vi "Get Test Library Path.vi"(11 "LUnit Test Suite Tests in":refnum<class "LUnit Test Suite Tests.lvclass">) -> (2 "project containing lvlib path":path, 3 "lvlib path":path)   [LabVIEW 2020, in "LUnit Test Suite Tests.lvclass"]
uses:
  LUnit Test Suite Tests.lvclass
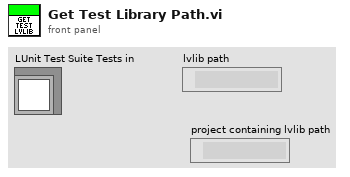
[diagram p1: front panel]
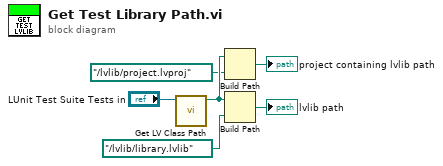
[diagram p0: block diagram]
diagram:
  n1 = call <vilib>:"Get LV Class Path.vi"("object"="LUnit Test Suite Tests in") -> ("class path"=w3:path)  [unwired: 9 in, 1 out]
  n2 = Build Path(base path=w3, name or relative path=path "../lvlib/project.lvproj") -> (appended path=→"project containing lvlib path":path)
  n3 = Build Path(base path=w3, name or relative path=path "../lvlib/library.lvlib") -> (appended path=→"lvlib path":path)
